vi "runReady.vi"(4 "FullRun? in":bool, 6 "Fault?":bool, 7 "Time in":dbl, 8 "error in (no error)":errorcluster, 9 "Actuators in":T1, 10 "State in":T2, 11 "RunType in":refnum<class "RunType.lvclass">) -> (0 "error out":errorcluster, 1 "Actuators out":T1, 2 "State out":T2, 3 "RunType out":refnum<class "RunType.lvclass">, 5 "FullRun? out":bool)   [LabVIEW 2018, in "ControlLibrary.lvlib" / "RunType.lvclass"]
uses:
  RunType.lvclass
  TypeDef_ControlState.ctl
  TypeDef_DigitalOuts.ctl
  TypeDef_RunParameters.ctl
  RunType.lvclass/RunType.ctl
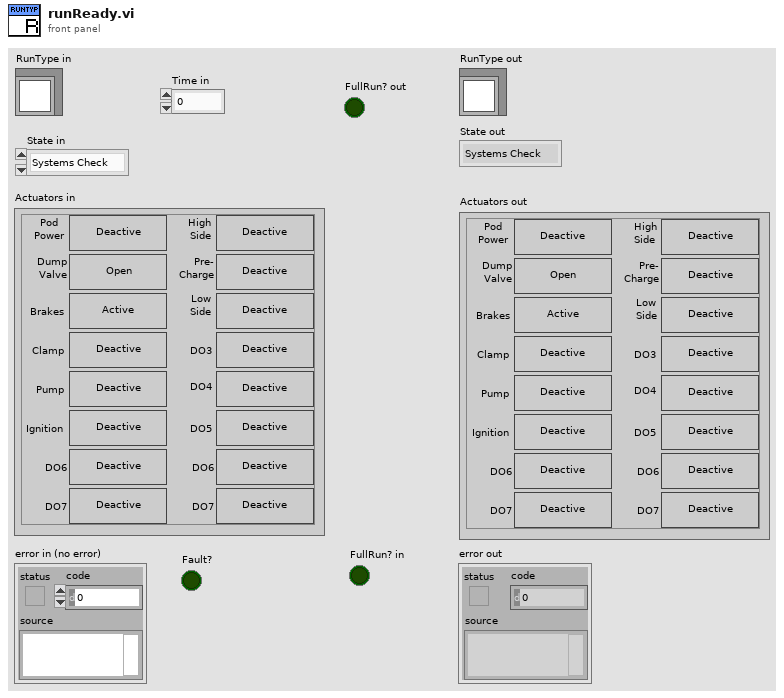
[diagram p1: front panel]
types:
  T1 = typedef "TypeDef_DigitalOuts.ctl" = cluster{"Pod Power":bool, "Dump Valve":bool, "Brakes":bool, "Clamp":bool, "Pump":bool, "Ignition":bool, "DO6":bool, "DO7":bool, "HighSide":bool, "Precharge":bool, "LowSide":bool, "DO3":bool, "DO4":bool, "DO5":bool, "DO62":bool, "DO72":bool}
  T2 = typedef "TypeDef_ControlState.ctl" = enum16{"Systems Check", "Idle", "Ready", "Pushing", "Coast", "Braking", "Fault", "Shutdown", "Service", "Precharge", "Blank"}
  T3 = typedef "TypeDef_RunParameters.ctl" = cluster{"Distance Threshold (ft)":dbl, "Time Threshold (s)":dbl, "Target (I16)":i16}
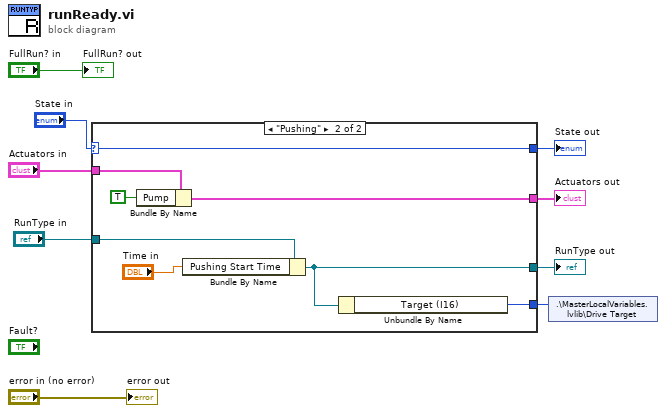
[diagram p0: block diagram]
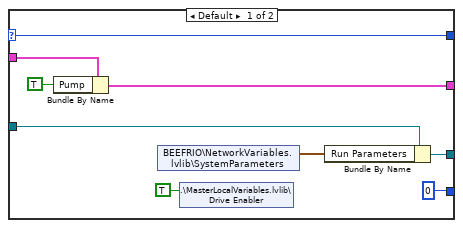
[diagram p2: hidden frame]
diagram:
  n1 = case shown="\"Pushing\"" "State in" {
    selector: "State in" -> [w18 w26]
    tunnel: [w18 w26] -> w6
    tunnel: "RunType in" -> [w13 w24]
    tunnel: [w17 w20] -> w7
    tunnel: [w15 w22] -> w2
    tunnel: "Actuators in" -> [w16 w23]
    tunnel: [i16 0 w19] -> w1
    frame Default {
      n2 = Bundle By Name(cluster=w16, "Pump"=TRUE ("Actuators.Pump")) -> (w15:T1)
      n3 = shared-variable "BEEFRIO\\NetworkVariables.lvlib\\SystemParameters"() -> (w14:T3)  [unwired: 1 in, 1 out]
      n4 = shared-variable ".\\MasterLocalVariables.lvlib\\Drive Enabler"(TRUE ("Drive Enabler")) -> ()  [unwired: 1 in, 1 out]
      n5 = Bundle By Name(cluster=w13, "Run Parameters"=w14) -> (w17:refnum<class "RunType.lvclass">)
    }
    frame "Pushing" {
      n6 = Bundle By Name(cluster=w23, "Pump"=TRUE ("Actuators.Pump")) -> (w22:T1)
      n7 = Bundle By Name(cluster=w24, "Pushing Start Time"="Time in") -> (w20:refnum<class "RunType.lvclass">)
      n8 = Unbundle By Name(w20) -> ("Target (I16)"=w19:i16)
    }
  }
  "RunType out" <- w7
  "State out" <- w6
  "Actuators out" <- w2
  n9 = shared-variable ".\\MasterLocalVariables.lvlib\\Drive Target"(w1) -> ()  [unwired: 1 in, 1 out]
  "error out" <- "error in (no error)"
  "FullRun? out" <- "FullRun? in"
